vi "Read formattedEvent.vi"(8 "error in (no error)":errorcluster, 11 "EventData in":refnum<class "EventData.lvclass">) -> (0 "error out":errorcluster, 2 "formattedEvent":string[](array[string]), 3 "EventData out":refnum<class "EventData.lvclass">)   [LabVIEW 2016, in "Event Logging.lvlib" / "EventData.lvclass"]
uses:
  EventData.lvclass
  EventData.lvclass/EventData.ctl
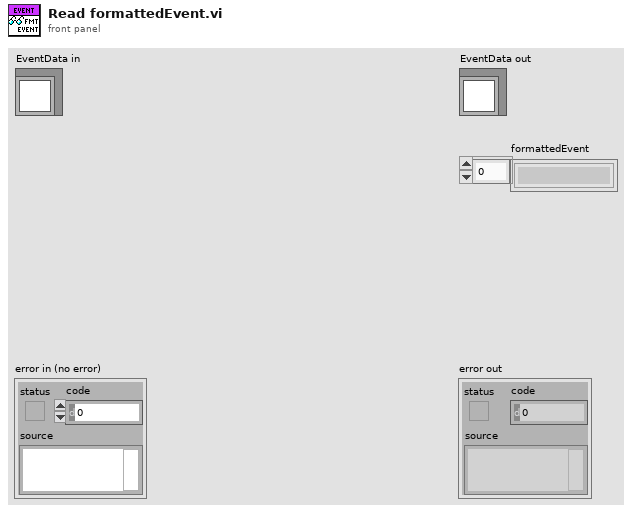
[diagram p1: front panel]
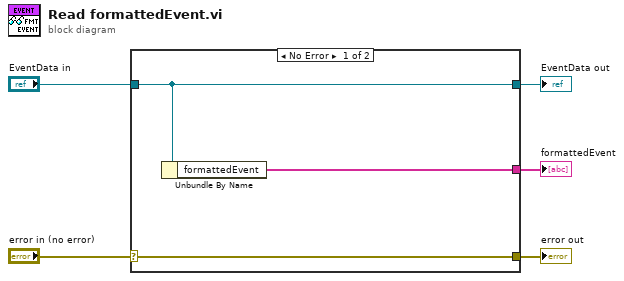
[diagram p0: block diagram]
diagram:
  n1 = case shown="No Error" "error in (no error)" {
    selector: "error in (no error)" -> [w8 w9]
    tunnel: [w8 w9] -> w4
    tunnel: [w7 w10] -> w2
    tunnel: "EventData in" -> [w7 w10]
    tunnel: [w6 _] -> w1
    frame No Error {
      n2 = Unbundle By Name(w7) -> ("formattedEvent"=w6:string[])
    }
    frame Error {
    }
  }
  "error out" <- w4
  "EventData out" <- w2
  "formattedEvent" <- w1
